vi "NMLWSD_Stability_Data_Collection RevA.vi"(0 "Instrumentation References":T3, 1 "Data Processing":T6, 2 "Tpass Shtr Open":bool, 3 "Log File":path=path "C:/Test/WSNM Stability/Log.txt", 5 "Serial Numbers & COM Ports":T4={"Serial Number"=["1"], "Active UUT COMs"=[]}, 7 "References":T5, 9 "UUT Input Parameters":T2 {"WL: NML Only" items=["Red Only", "IR"]; "FW inTest" items=["WSD Board", "NML Board"]}, 11 "Error In":errorcluster, 12 "Data Results In":T7 {"All Results In" format="%8_4g"}, 13 "Shtr Ctrl Close (s)":dbl=6.0 max=60.0 format="%.3f") -> (4 "Data Results Out":T8 {"All Results Out" format="%8_4g"}, 8 "Data Time":timestamp, 10 "Shtr Ref Time":timestamp, 15 "Error Out":errorcluster)   [LabVIEW 2017]
uses:
  C:/Program Files (x86)/Newport/Newport USB Driver/Bin/UsbDllWrap.dll
  Program Files (x86)/Newport/Newport USB Driver/Bin/UsbDllWrap.dll
  <vilib>/Analysis/baseanly.llb/Mean (DBL).vi
  <vilib>/Utility/file.llb/Write Delimited Spreadsheet (string).vi
  <vilib>/Analysis/NI_AALBase.lvlib
panel:
  in  "Tab Control":T1(tab)
  out "Error Log Msg":string
  out "Timeout":bool
  out "Data Errors":bool
  out "Module Errors":bool[](array[boolean])
  out "Msg":string="\n\r" caption="Status"
  out "Shtr Open":bool
  out "Shtr Close":bool
  out "read buffer":string
  out "MCU Data":dbl[](array[numeric]) format="%#_5p"
  out "System Data":dbl[](array[numeric]) format="%#_5p"
  out "UUT Download Buffer":string
  out "UUT Count":i32=1
  out "Bytes Rcvd":u32
  out "DateS":string caption="Date"
  out "TimeS":string caption="Time"
  out "MCUTrue":bool[][](array[boolean])
  out "SysTrue":bool[][](array[boolean])
  out "MCUCheck":string[][](array[string])
  out "SysCheck":string[][](array[string])
  out "Points":i32[](array[numeric])
  out "All Results Out":dbl[][][](array[numeric]) format="%8_4g"
  out "MCU Data Array":dbl[][](array[numeric])
  out "System Data Array":dbl[][](array[numeric])
  out "Module Error":refnum<vi>
  out "Read Buffer":refnum<vi>
  out "Error Log":refnum<vi>
  out "Data Error":refnum<vi>
  out "TimeOut Error":refnum<vi>
  out "Status Msg":refnum<vi>
  out "Shutter Closed":refnum<vi>
  out "Shutter Opened":refnum<vi>
  # "Indicators Passed To Calling VI via Control RefNum"
  # "Indicators With Data to be Passed to Calling VI Directly But Grouped Into Single Cluster"
  # "Indicators Passed to Calling VI Directly"
  # "Indicators Used To Store & Process Temporary Data for Each UUT"
  # "Indicators That Provide Information Not Necessary for Calling VI"
  # "Indicators Replicated in \"Data Results Out\" Output Cluster To Be Passed to Calling VI Via RefNum"
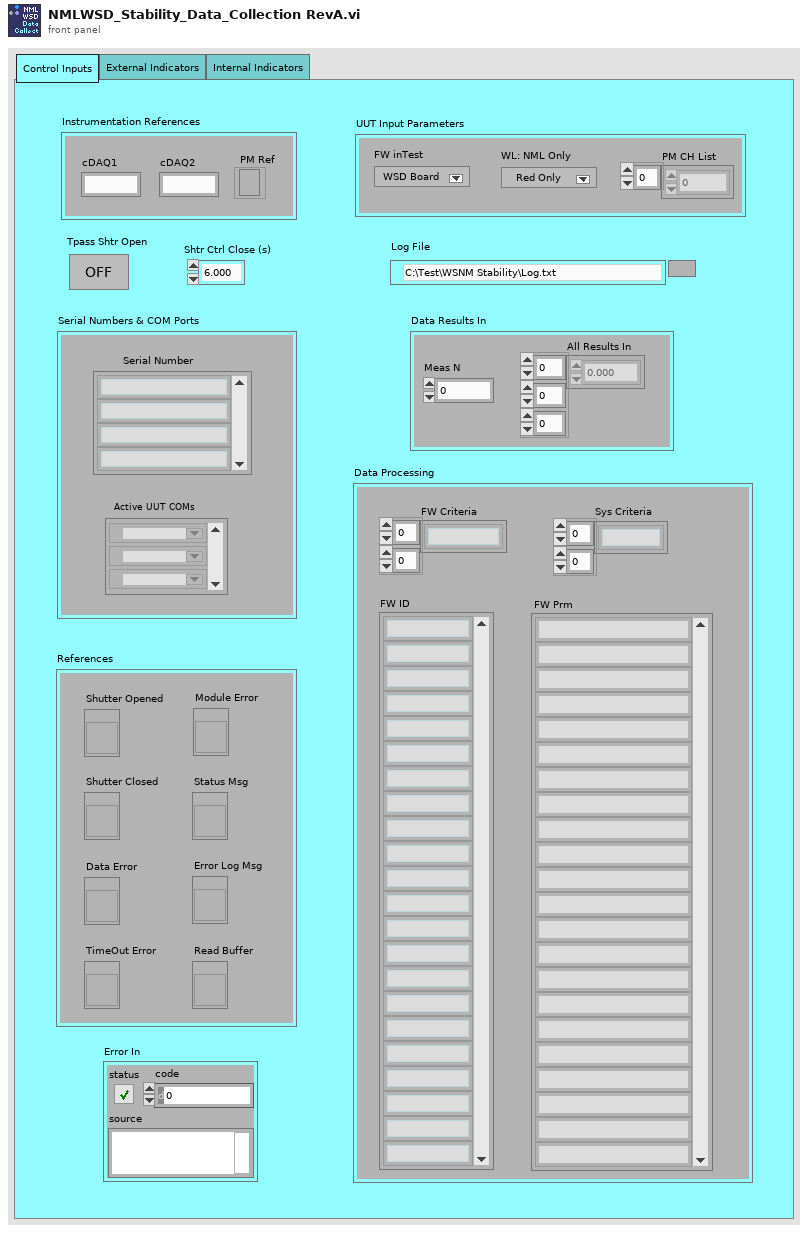
[diagram p1: front panel]
types:
  T1 = enum32{"Control Inputs", "External Indicators", "Internal Indicators"}
  T2 = cluster{"FW inTest":u16, "WL: NML Only":i32, "PM CH List":i32[]}
  T3 = cluster{"cDAQ1":string, "cDAQ2":string, "PM Ref":refnum<k24>}
  T4 = cluster{"Serial Number":string[], "Active UUT COMs":refnum<visa-resource-name>[]}
  T5 = cluster{"Shutter Opened":refnum<vi>, "Shutter Closed":refnum<vi>, "Status Msg":refnum<vi>, "TimeOut Error":refnum<vi>, "Data Error":refnum<vi>, "Error Log Msg":refnum<vi>, "Read Buffer":refnum<vi>, "Module Error":refnum<vi>}
  T6 = cluster{"FW Prm":string[], "FW ID":string[], "FW Criteria":string[][], "Sys Criteria":string[][]}
  T7 = cluster{"Meas N":i32, "All Results In":dbl[][][]}
  T8 = cluster{"MCUTrue":bool[][], "SysTrue":bool[][], "MCUCheck":string[][], "SysCheck":string[][], "Points":i32[], "All Results Out ":dbl[][][], "MCU Data Array":dbl[][], "System Data Array":dbl[][]}
  T9 = cluster{"MCUTrue":bool[][], "SysTrue":bool[][], "MCUCheck":string[][], "SysCheck":string[][], "Points":i32[], "All Results ":dbl[][][], "MCU Data Array":dbl[][], "System Data Array":dbl[][]}
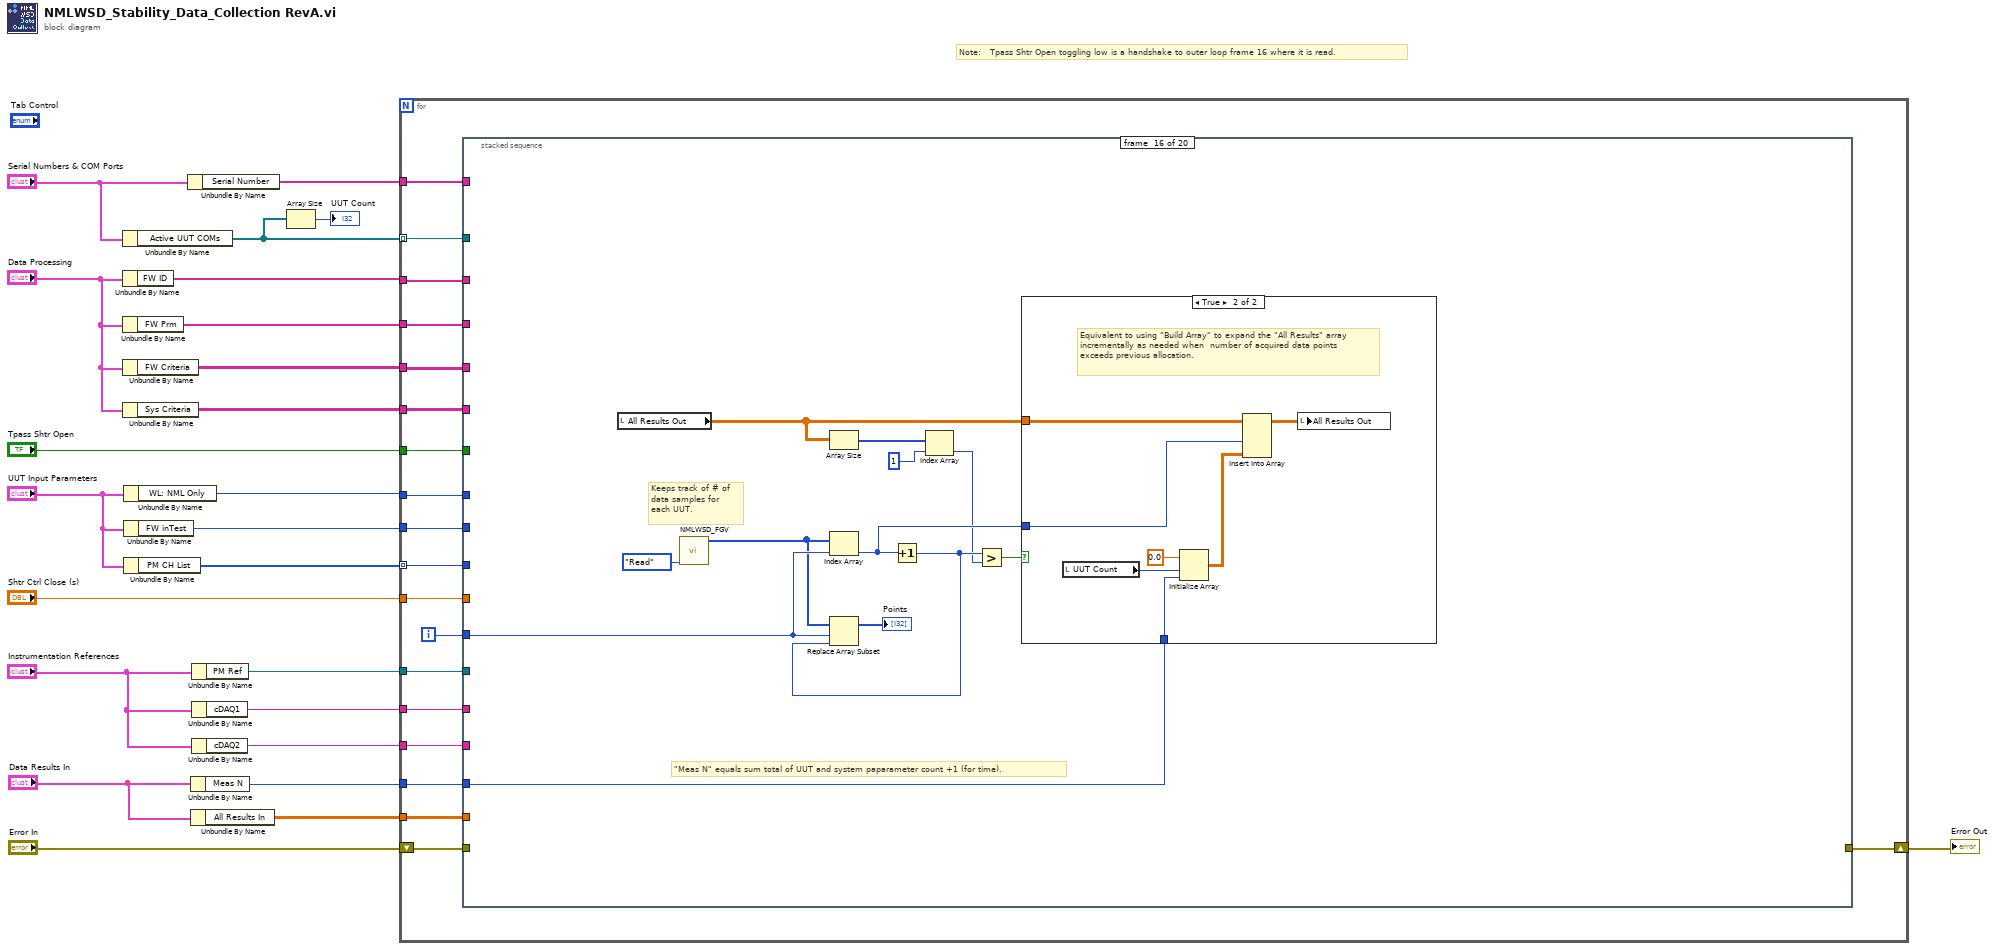
[diagram p0: block diagram]
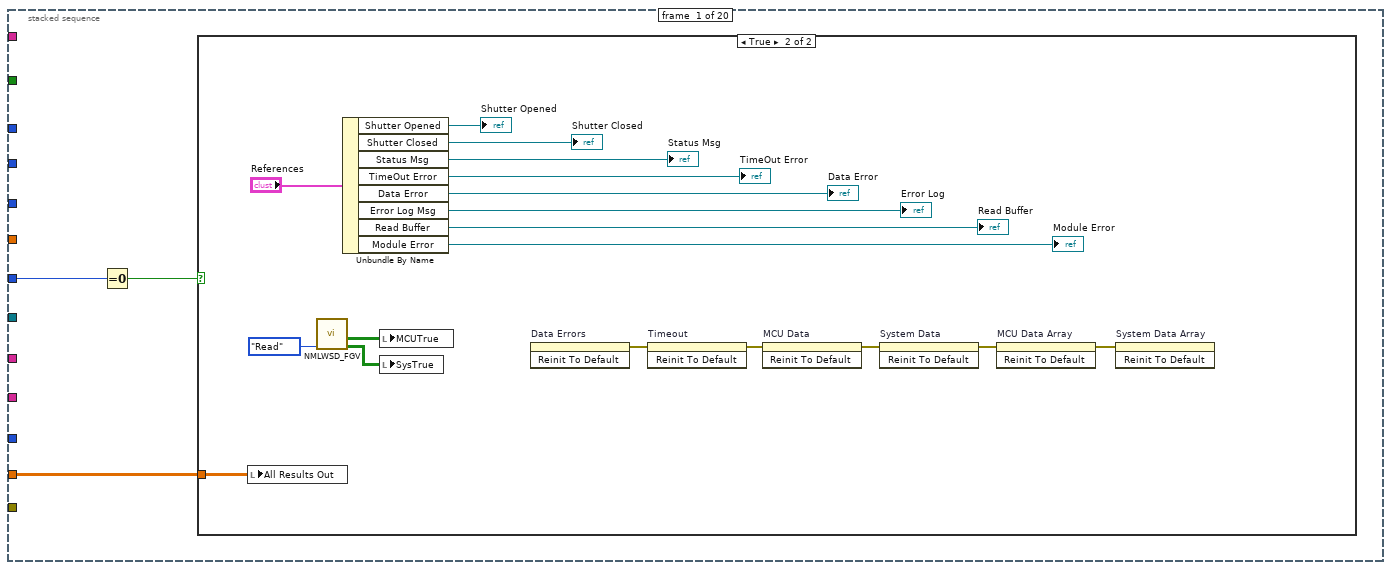
[diagram p2: hidden frame]
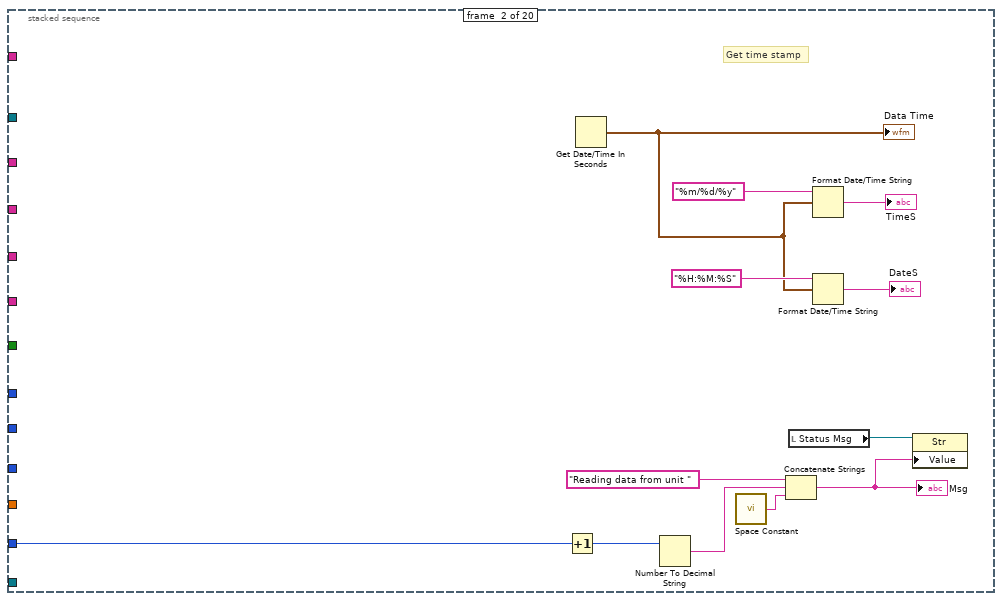
[diagram p4: hidden frame]
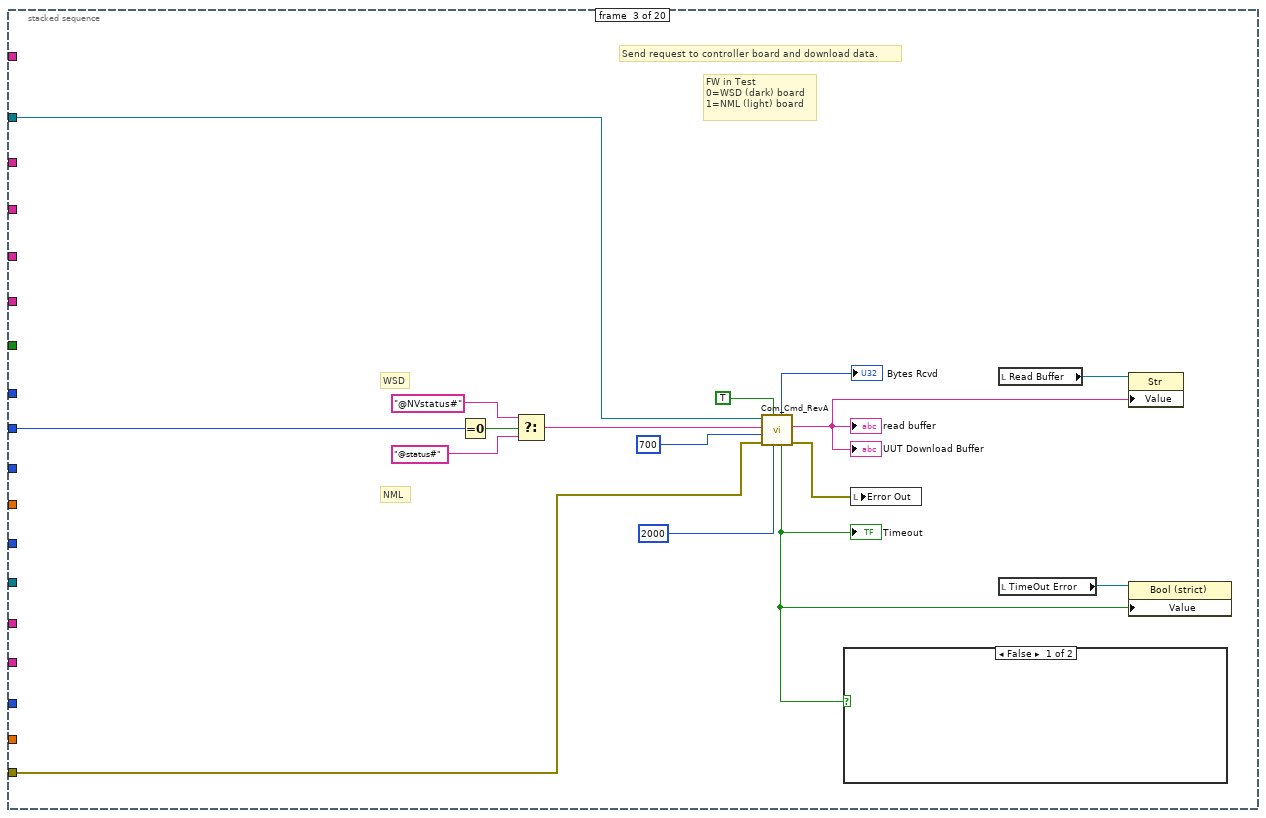
[diagram p5: hidden frame]
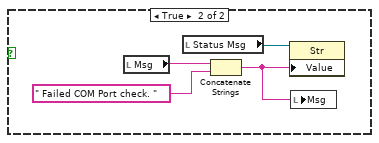
[diagram p6: hidden frame]
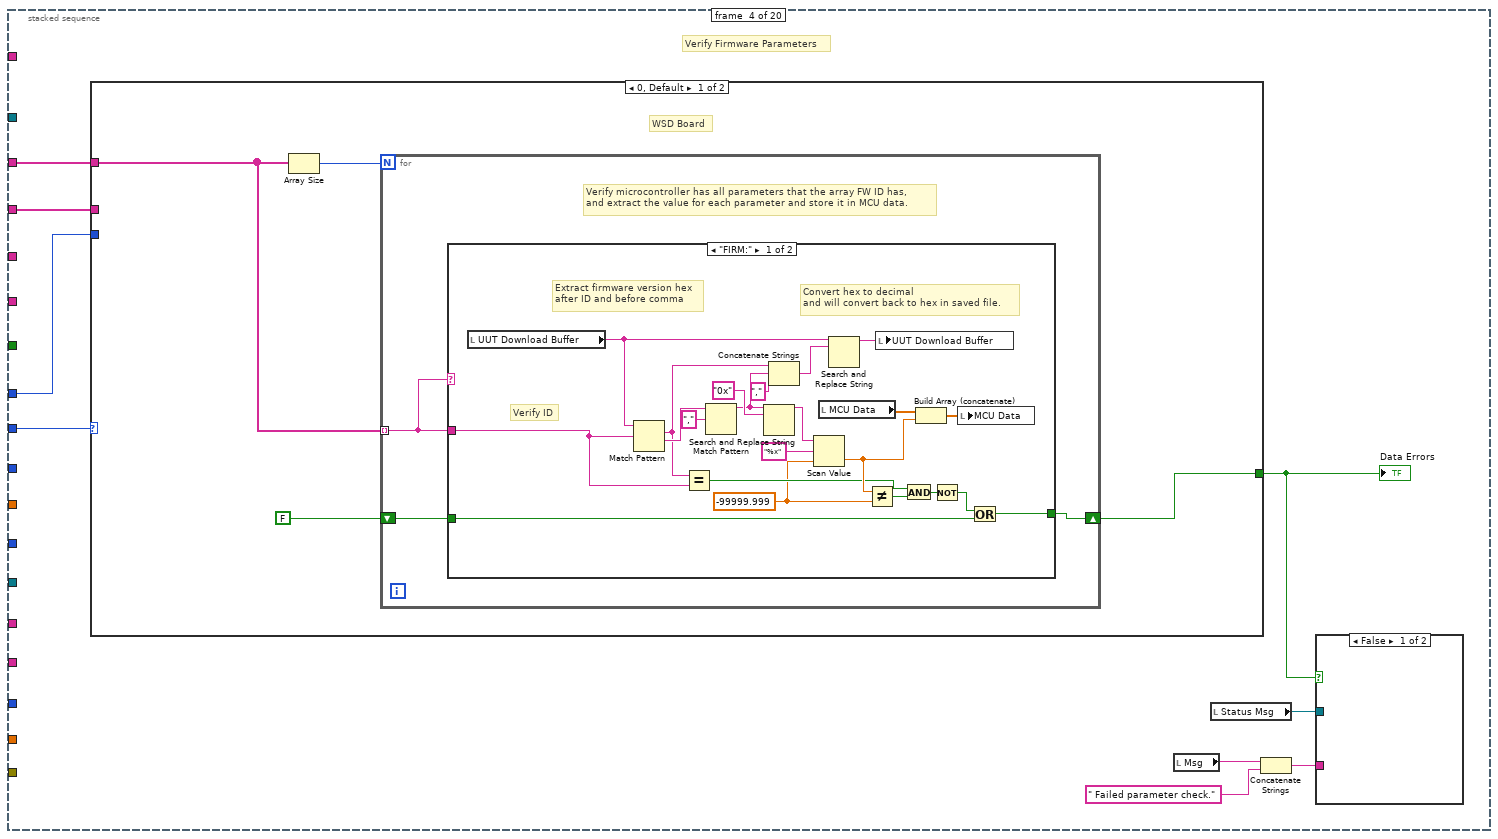
[diagram p7: hidden frame]
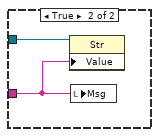
[diagram p8: hidden frame]
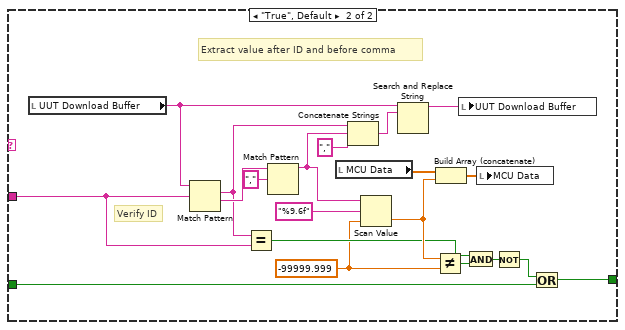
[diagram p9: hidden frame]
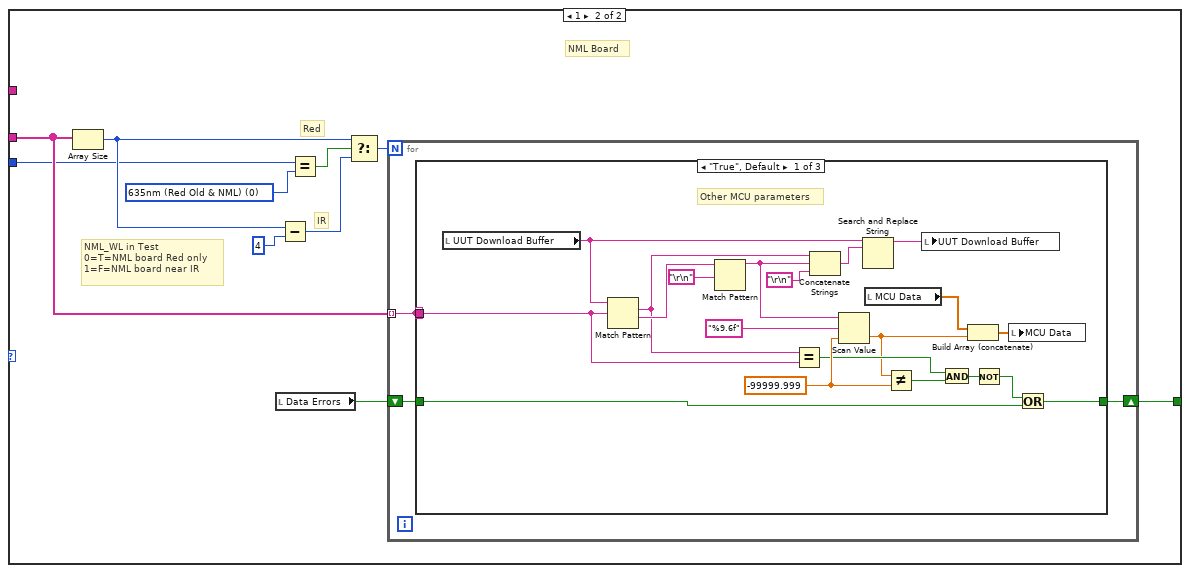
[diagram p10: hidden frame]
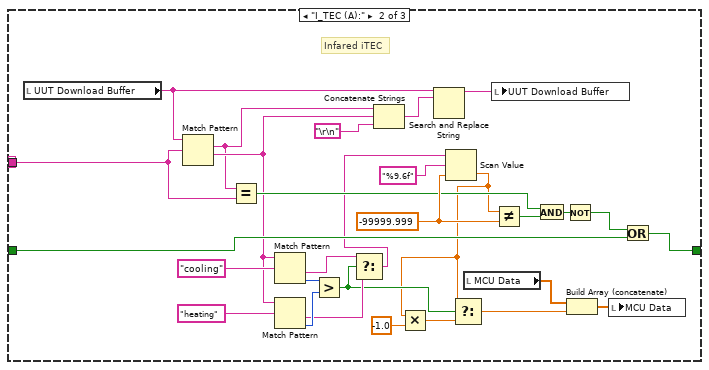
[diagram p11: hidden frame]
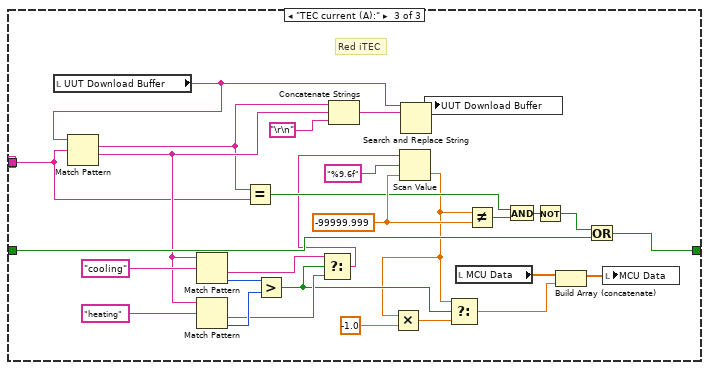
[diagram p12: hidden frame]
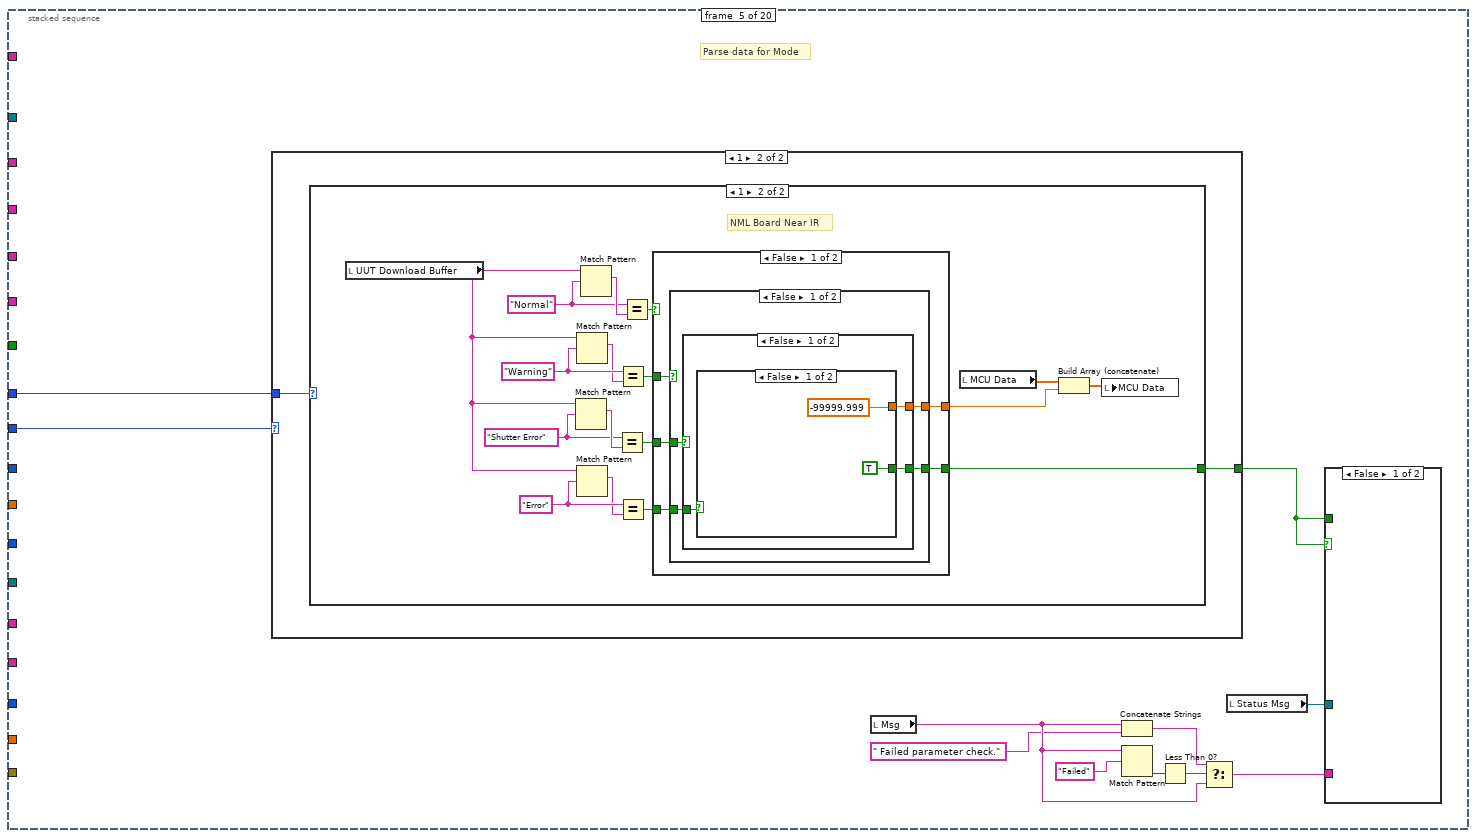
[diagram p13: hidden frame]
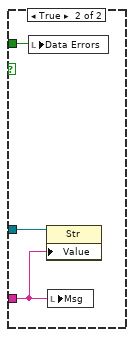
[diagram p14: hidden frame]
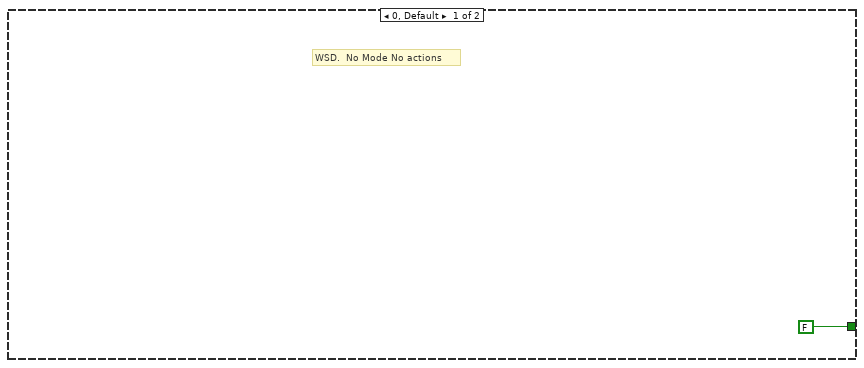
[diagram p15: hidden frame]
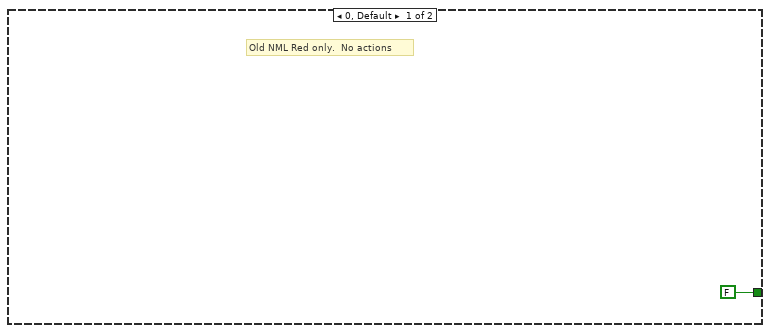
[diagram p16: hidden frame]
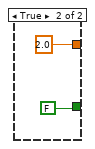
[diagram p17: hidden frame]
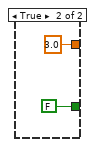
[diagram p18: hidden frame]
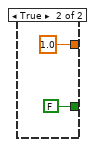
[diagram p19: hidden frame]
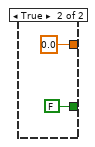
[diagram p20: hidden frame]
diagram:
  # "Note:   Tpass Shtr Open toggling low is a handshake to outer loop frame 16 where it is read."
  n1 = Unbundle By Name("Serial Numbers & COM Ports") -> ("Active UUT COMs"=w13:refnum<visa-resource-name>[])
  n2 = Unbundle By Name("Data Processing") -> ("FW ID"=w12:string[])
  n3 = Unbundle By Name("Data Processing") -> ("FW Prm"=w11:string[])
  n4 = Unbundle By Name("Data Processing") -> ("FW Criteria"=w10:string[][])
  n5 = Unbundle By Name("Data Processing") -> ("Sys Criteria"=w8:string[][])
  n6 = Unbundle By Name("UUT Input Parameters") -> ("WL: NML Only"=w21:i32)
  n7 = Unbundle By Name("UUT Input Parameters") -> ("FW inTest"=w20:u16)
  n8 = Unbundle By Name("UUT Input Parameters") -> ("PM CH List"=w1:i32[])
  n9 = Unbundle By Name("Serial Numbers & COM Ports") -> ("Serial Number"=w14:string[])
  n10 = Unbundle By Name("Data Results In") -> ("Meas N"=w7:i32)
  n11 = Unbundle By Name("Data Results In") -> ("All Results In"=w5:dbl[][][])
  n12 = Unbundle By Name("Instrumentation References") -> ("PM Ref"=w19:refnum<k24>)
  n13 = Unbundle By Name("Instrumentation References") -> ("cDAQ1"=w17:string)
  n14 = Unbundle By Name("Instrumentation References") -> ("cDAQ2"=w16:string)
  n15 = Array Size(array=w13) -> (size(s)=→"UUT Count":i32)
  n16 = for {
    tunnel: w13 -> [w42] mode=indexing
    tunnel: w19 -> [w41]
    tunnel: "Tpass Shtr Open" -> [w40]
    tunnel: w20 -> [w39]
    tunnel: w21 -> [w38]
    tunnel: "Shtr Ctrl Close (s)" -> [w37]
    tunnel: w17 -> [w36]
    tunnel: w16 -> [w35]
    tunnel: w12 -> [w34]
    tunnel: w7 -> [w33]
    tunnel: w14 -> [w32]
    tunnel: w8 -> [w31]
    tunnel: w10 -> [w30]
    tunnel: w11 -> [w29]
    tunnel: w5 -> [w28]
    shift-right: [w26] -> w3
    shift-left: "Error In" -> [w27]
    tunnel: w1 -> [w25] mode=indexing
    i -> [w43]
    n17 = stacked-sequence {
      tunnel: w43 -> [w45 w65 _ _ _ _ _ w412 _ _ _ _ _ w517 w587 w698 w720 w730 w771 w795]
      tunnel: w42 -> [_ _ w85 _ _ _ _ _ _ _ _ _ _ _ _ _ _ _ _ _]
      tunnel: w41 -> [_ _ _ _ _ _ _ _ _ w461 _ _ _ _ w593 _ _ _ _ _]
      tunnel: w40 -> [_ _ _ _ _ _ _ _ _ _ _ _ _ _ w592 _ _ _ _ _]
      tunnel: w39 -> [_ _ w81 w105 w258 w315 w372 _ _ _ _ _ _ _ _ _ _ _ _ _]
      tunnel: w38 -> [_ _ _ w98 w257 w314 w371 _ _ _ _ _ _ _ _ _ _ _ _ _]
      tunnel: w37 -> [_ _ _ _ _ _ _ _ _ _ _ _ _ _ w591 _ _ _ _ _]
      tunnel: w36 -> [_ _ _ _ _ _ _ _ _ _ _ w489 _ w516 w590 _ _ _ _ _]
      tunnel: w35 -> [_ _ _ _ _ _ _ _ _ _ _ _ _ w515 w589 _ _ _ _ _]
      tunnel: w34 -> [_ _ _ w104 _ _ _ _ _ _ _ _ _ _ _ _ _ _ _ _]
      tunnel: w33 -> [_ _ _ _ _ _ _ _ _ _ _ _ _ _ _ w697 _ _ _ _]
      tunnel: w32 -> [_ _ _ _ _ _ _ w410 _ _ _ _ _ _ _ _ _ _ _ _]
      tunnel: w31 -> [_ _ _ _ _ _ _ _ _ _ _ _ _ _ _ _ _ w729 _ _]
      tunnel: w30 -> [_ _ _ _ _ _ _ _ _ _ _ _ _ _ _ _ _ w728 _ _]
      tunnel: w29 -> [_ _ _ w99 _ _ _ _ _ _ _ _ _ _ _ _ _ _ _ _]
      tunnel: w28 -> [w44 _ _ _ _ _ _ _ _ _ _ _ _ _ _ _ _ _ _ _]
      tunnel: w27 -> [_ _ w78 _ _ _ _ _ _ _ _ _ _ _ _ _ _ _ _ _]
      tunnel: [_ _ _ _ _ _ _ _ _ w460 _ _ _ _ _ _ _ _ _ _] -> w26
      tunnel: w25 -> [_ _ _ _ _ _ _ _ _ w459 _ _ _ _ w588 _ _ _ _ _]
      frame #0 {
        n18 = Equal To 0?(x=w45) -> (x = 0?=w46:bool)
        n19 = case shown="True" w46 {
          tunnel: w44 -> [_ w52]
          frame False {
          }
          frame True {
            n20 = local write "All Results Out"(w52) -> ()
            n21 = call "NMLWSD_FGV.vi"("Action"=enum16{"Initialize", "Read", "Write"}."Read") -> ("SysTrue"=w51:bool[][], "MCUTrue"=w50:bool[][])  [unwired: 8 in, 1 out]
            n22 = Unbundle By Name("References") -> ("Shutter Opened"=→"Shutter Opened":refnum<vi>, "Shutter Closed"=→"Shutter Closed":refnum<vi>, "Status Msg"=→"Status Msg":refnum<vi>, "TimeOut Error"=→"TimeOut Error":refnum<vi>, "Data Error"=→"Data Error":refnum<vi>, "Error Log Msg"=→"Error Log":refnum<vi>, "Read Buffer"=→"Read Buffer":refnum<vi>, "Module Error"=→"Module Error":refnum<vi>)
            n23 = local write "MCUTrue"(w50) -> ()
            n24 = local write "SysTrue"(w51) -> ()
            n25 = invoke on="Data Errors" class="Bool (strict)" method="Reinit To Default"() -> (error out=w63:errorcluster)  [unwired: 3 in, 2 out]
            n26 = invoke on="Timeout" class="Bool (strict)" method="Reinit To Default"(error in=w63) -> (error out=w62:errorcluster)  [unwired: 2 in, 2 out]
            n27 = invoke on="MCU Data" class="Arr (strict)" method="Reinit To Default"(error in=w62) -> (error out=w64:errorcluster)  [unwired: 2 in, 2 out]
            n28 = invoke on="System Data" class="Arr (strict)" method="Reinit To Default"(error in=w64) -> (error out=w48:errorcluster)  [unwired: 2 in, 2 out]
            n29 = invoke on="MCU Data Array" class="Arr (strict)" method="Reinit To Default"(error in=w48) -> (error out=w47:errorcluster)  [unwired: 2 in, 2 out]
            n30 = invoke on="System Data Array" class="Arr (strict)" method="Reinit To Default"(error in=w47) -> ()  [unwired: 2 in, 3 out]
          }
        }
      }
      frame #1 {
        # "Get time stamp"
        n31 = Increment(x=w65) -> (x+1=w71:i32)
        n32 = Get Date/Time In Seconds() -> (seconds since 1Jan1904=w72:timestamp)
        "Data Time" <- w72
        n33 = Number To Decimal String(number=w71) -> (decimal integer string=w70:string)  [unwired: 1 in]
        n34 = call <vilib>:"Space Constant.vi"() -> ("String"=w68:string)
        n35 = Concatenate Strings("Reading data from unit " ("Msg"), w70, w68) -> (w69:string)
        "Msg" <- w69
        n36 = local read "Status Msg"() -> (w67:refnum<vi>)
        n37 = Format Date/Time String(time format string (%c)="%m/%d/%y", seconds (now)=w72) -> (date/time string=→"TimeS":string)  [unwired: 1 in]
        n38 = Format Date/Time String(time format string (%c)="%H:%M:%S", seconds (now)=w72) -> (date/time string=→"DateS":string)  [unwired: 1 in]
        n39 = property class="Str"(reference=w67, "Value"=w69) -> ()  [unwired: 1 in, 2 out]
      }
      frame #2 {
        # "NML"
        # "WSD"
        # "FW in Test\n0=WSD (dark) board\n1=NML (light) board"
        # "Send request to controller board and download data."
        n40 = Equal To 0?(x=w81) -> (x = 0?=w86:bool)
        n41 = Select(t="@NVstatus#" ("string"), s=w86, f="@status#" ("string")) -> (s? t:f=w89:string)
        n42 = call "Com_Cmd_RevA.vi"("Timeout"=2000, "Query"=TRUE, "error in"=w78, "Delay, ms"=u32 700, "write buffer"=w89, "VISA"=w85) -> ("error out"=w77:errorcluster, "read buffer"=w83:string, "Timeout"=w84:bool, "return count"=→"Bytes Rcvd":u32)  [unwired: 2 out]
        "UUT Download Buffer" <- w83
        "Timeout" <- w84
        "read buffer" <- w83
        n43 = case shown="False" w84 {
          frame False {
          }
          frame True {
            n44 = local read "Msg"() -> (w96:string)
            n45 = local read "Status Msg"() -> (w93:refnum<vi>)
            n46 = Concatenate Strings(w96, " Failed COM Port check. " ("string")) -> (w94:string)
            n47 = property class="Str"(reference=w93, "Value"=w94) -> ()  [unwired: 1 in, 2 out]
            n48 = local write "Msg"(w94) -> ()
          }
        }
        n49 = local write "Error Out"(w77) -> ()
        n50 = local read "Read Buffer"() -> (w79:refnum<vi>)
        n51 = local read "TimeOut Error"() -> (w80:refnum<vi>)
        n52 = property class="Str"(reference=w79, "Value"=w83) -> ()  [unwired: 1 in, 2 out]
        n53 = property class="Bool (strict)"(reference=w80, "Value"=w84) -> ()  [unwired: 1 in, 2 out]
      }
      frame #3 {
        # "Verify Firmware Parameters"
        n54 = case shown="0, Default" w105 {
          tunnel: w104 -> [w109 _]
          tunnel: [w108 w159] -> w103
          tunnel: w99 -> [_ w158]
          tunnel: w98 -> [_ w157]
          frame 0, Default {
            # "WSD Board"
            n55 = Array Size(array=w109) -> (size(s)=w110:i32)
            n56 = for {
              N: w110 -> [_]
              shift-right: [w113] -> w108
              shift-left: FALSE ("Data Err") -> [w114]
              tunnel: w109 -> [w112] mode=indexing
              # "Verify microcontroller has all parameters that the array FW ID has,\nand extract the value for each parameter and store it in MCU data."
              n57 = case shown="\"FIRM:\"" w112 {
                tunnel: w112 -> [w115 w137]
                tunnel: w114 -> [w125 w156]
                tunnel: [w124 w155] -> w113
                frame "FIRM:" {
                  w129 = -99999.999 ("default (0 dbl)")
                  # "Convert hex to decimal\nand will convert back to hex in saved file."
                  # "Extract firmware version hex\nafter ID and before comma"
                  # "Verify ID"
                  n58 = local read "UUT Download Buffer"() -> (w119:string)
                  n59 = Match Pattern(string=w119, regular expression=w115) -> (match substring=w116:string, after substring=w127:string)  [unwired: 1 in, 2 out]
                  n60 = Equal?(x=w116, y=w115) -> (x = y?=w131:bool)
                  n61 = Match Pattern(string=w127, regular expression=",") -> (before substring=w121:string)  [unwired: 1 in, 3 out]
                  n62 = Search and Replace String(input string=w121, search string="0x") -> (result string=w122:string)  [unwired: 6 in, 3 out]
                  n63 = Concatenate Strings(w116, w121, "," ("string")) -> (w118:string)
                  n64 = Scan Value(string=w122, format string="%x", default (0 dbl)=w129) -> (value=w134:dbl)  [unwired: 1 out]
                  n65 = local read "MCU Data"() -> (w132:dbl[])
                  n66 = Search and Replace String(input string=w119, search string=w118) -> (result string=w117:string)  [unwired: 6 in, 3 out]
                  n67 = Not Equal?(x=w134, y=w129) -> (x != y?=w130:bool)
                  n68 = local write "UUT Download Buffer"(w117) -> ()
                  n69 = And(x=w131, y=w130) -> (x .and. y?=w135:bool)
                  n70 = Build Array (concatenate)(w132, w134) -> (w133:dbl[])
                  n71 = Not(x=w135) -> (.not. x?=w136:bool)
                  n72 = local write "MCU Data"(w133) -> ()
                  n73 = Or(x=w136, y=w125) -> (x .or. y?=w124:bool)
                }
                frame "True", Default {
                  w147 = -99999.999 ("default (0 dbl)")
                  # "Extract value after ID and before comma"
                  # "Verify ID"
                  n74 = local read "UUT Download Buffer"() -> (w141:string)
                  n75 = Match Pattern(string=w141, regular expression=w137) -> (match substring=w138:string, after substring=w145:string)  [unwired: 1 in, 2 out]
                  n76 = Equal?(x=w138, y=w137) -> (x = y?=w149:bool)
                  n77 = Match Pattern(string=w145, regular expression=",") -> (before substring=w142:string)  [unwired: 1 in, 3 out]
                  n78 = local read "MCU Data"() -> (w150:dbl[])
                  n79 = Concatenate Strings(w138, w142, "," ("string")) -> (w140:string)
                  n80 = Scan Value(string=w142, format string="%9.6f", default (0 dbl)=w147) -> (value=w152:dbl)  [unwired: 1 out]
                  n81 = Search and Replace String(input string=w141, search string=w140) -> (result string=w139:string)  [unwired: 6 in, 3 out]
                  n82 = Not Equal?(x=w152, y=w147) -> (x != y?=w148:bool)
                  n83 = Build Array (concatenate)(w150, w152) -> (w151:dbl[])
                  n84 = local write "UUT Download Buffer"(w139) -> ()
                  n85 = And(x=w149, y=w148) -> (x .and. y?=w153:bool)
                  n86 = local write "MCU Data"(w151) -> ()
                  n87 = Not(x=w153) -> (.not. x?=w154:bool)
                  n88 = Or(x=w154, y=w156) -> (x .or. y?=w155:bool)
                }
              }
            }
          }
          frame 1 {
            w161 = 0 items=["635nm (Red Old & NML)", "Red-780-850nm (IR NewNML FW)", "Mix NML FW"] ("Color")
            # "NML Board"
            # "NML_WL in Test\n0=T=NML board Red only\n1=F=NML board near IR"
            # "IR"
            # "Red"
            n89 = Array Size(array=w158) -> (size(s)=w164:i32)
            n90 = local read "Data Errors"() -> (w160:bool)
            n91 = Subtract(x=w164, y=4) -> (x-y=w162:i32)
            n92 = Equal?(x=w157, y=w161) -> (x = y?=w166:bool)
            n93 = Select(t=w164, s=w166, f=w162) -> (s? t:f=w165:i32)
            n94 = for {
              N: w165 -> [_]
              tunnel: w158 -> [w167] mode=indexing
              shift-right: [w168] -> w159
              shift-left: w160 -> [w169]
              n95 = case shown="\"True\", Default" w167 {
                tunnel: w169 -> [w180 w210 w239]
                tunnel: [w179 w209 w238] -> w168
                tunnel: w167 -> [w171 w190 w220]
                frame "True", Default {
                  w188 = -99999.999 ("default (0 dbl)")
                  # "Other MCU parameters"
                  n96 = local read "UUT Download Buffer"() -> (w170:string)
                  n97 = Match Pattern(string=w170, regular expression=w171) -> (match substring=w172:string, after substring=w177:string)  [unwired: 1 in, 2 out]
                  n98 = Match Pattern(string=w177, regular expression="\r\n") -> (before substring=w175:string)  [unwired: 1 in, 3 out]
                  n99 = Equal?(x=w172, y=w171) -> (x = y?=w186:bool)
                  n100 = Concatenate Strings(w172, w175, "\r\n") -> (w174:string)
                  n101 = Scan Value(string=w175, format string="%9.6f", default (0 dbl)=w188) -> (value=w183:dbl)  [unwired: 1 out]
                  n102 = Search and Replace String(input string=w170, search string=w174) -> (result string=w173:string)  [unwired: 6 in, 3 out]
                  n103 = local read "MCU Data"() -> (w185:dbl[])
                  n104 = Not Equal?(x=w183, y=w188) -> (x != y?=w187:bool)
                  n105 = local write "UUT Download Buffer"(w173) -> ()
                  n106 = And(x=w186, y=w187) -> (x .and. y?=w182:bool)
                  n107 = Build Array (concatenate)(w185, w183) -> (w184:dbl[])
                  n108 = Not(x=w182) -> (.not. x?=w181:bool)
                  n109 = local write "MCU Data"(w184) -> ()
                  n110 = Or(x=w181, y=w180) -> (x .or. y?=w179:bool)
                }
                frame "I_TEC (A):" {
                  w217 = -99999.999 ("default (0 dbl)")
                  # "Infared iTEC"
                  n111 = local read "UUT Download Buffer"() -> (w194:string)
                  n112 = Match Pattern(string=w194, regular expression=w190) -> (match substring=w191:string, after substring=w192:string)  [unwired: 1 in, 2 out]
                  n113 = Equal?(x=w191, y=w190) -> (x = y?=w215:bool)
                  n114 = Match Pattern(string=w192, regular expression="cooling") -> (after substring=w204:string, offset past match=w206:i32)  [unwired: 1 in, 2 out]
                  n115 = Match Pattern(string=w192, regular expression="heating") -> (after substring=w203:string, offset past match=w205:i32)  [unwired: 1 in, 2 out]
                  n116 = Greater?(x=w206, y=w205) -> (0:w202:bool)
                  n117 = Select(t=w204, s=w202, f=w203) -> (s? t:f=w193:string)
                  n118 = Concatenate Strings(w191, w192, "\r\n") -> (w197:string)
                  n119 = Search and Replace String(input string=w194, search string=w197) -> (result string=w196:string)  [unwired: 6 in, 3 out]
                  n120 = Scan Value(string=w193, format string="%9.6f", default (0 dbl)=w217) -> (value=w199:dbl)  [unwired: 1 out]
                  n121 = Multiply(x=w199, y=-1.0) -> (x*y=w200:dbl)
                  n122 = Select(t=w199, s=w202, f=w200) -> (s? t:f=w198:dbl)
                  n123 = local read "MCU Data"() -> (w214:dbl[])
                  n124 = local write "UUT Download Buffer"(w196) -> ()
                  n125 = Not Equal?(x=w199, y=w217) -> (x != y?=w216:bool)
                  n126 = And(x=w215, y=w216) -> (x .and. y?=w212:bool)
                  n127 = Not(x=w212) -> (.not. x?=w211:bool)
                  n128 = Build Array (concatenate)(w214, w198) -> (w213:dbl[])
                  n129 = local write "MCU Data"(w213) -> ()
                  n130 = Or(x=w211, y=w210) -> (x .or. y?=w209:bool)
                }
                frame "TEC current (A):" {
                  w246 = -99999.999 ("default (0 dbl)")
                  # "Red iTEC"
                  n131 = local read "UUT Download Buffer"() -> (w222:string)
                  n132 = Match Pattern(string=w222, regular expression=w220) -> (match substring=w219:string, after substring=w221:string)  [unwired: 1 in, 2 out]
                  n133 = Match Pattern(string=w221, regular expression="cooling") -> (after substring=w233:string, offset past match=w235:i32)  [unwired: 1 in, 2 out]
                  n134 = Match Pattern(string=w221, regular expression="heating") -> (after substring=w232:string, offset past match=w234:i32)  [unwired: 1 in, 2 out]
                  n135 = Equal?(x=w219, y=w220) -> (x = y?=w244:bool)
                  n136 = Greater?(x=w235, y=w234) -> (0:w230:bool)
                  n137 = Select(t=w233, s=w230, f=w232) -> (s? t:f=w231:string)
                  n138 = Concatenate Strings(w219, w221, "\r\n") -> (w225:string)
                  n139 = Scan Value(string=w231, format string="%9.6f", default (0 dbl)=w246) -> (value=w227:dbl)  [unwired: 1 out]
                  n140 = Multiply(x=w227, y=-1.0) -> (x*y=w228:dbl)
                  n141 = Search and Replace String(input string=w222, search string=w225) -> (result string=w224:string)  [unwired: 6 in, 3 out]
                  n142 = local write "UUT Download Buffer"(w224) -> ()
                  n143 = Select(t=w227, s=w230, f=w228) -> (s? t:f=w226:dbl)
                  n144 = local read "MCU Data"() -> (w243:dbl[])
                  n145 = Not Equal?(x=w227, y=w246) -> (x != y?=w245:bool)
                  n146 = And(x=w244, y=w245) -> (x .and. y?=w241:bool)
                  n147 = Not(x=w241) -> (.not. x?=w240:bool)
                  n148 = Build Array (concatenate)(w243, w226) -> (w242:dbl[])
                  n149 = Or(x=w240, y=w239) -> (x .or. y?=w238:bool)
                  n150 = local write "MCU Data"(w242) -> ()
                }
              }
            }
          }
        }
        "Data Errors" <- w103
        n151 = local read "Msg"() -> (w102:string)
        n152 = local read "Status Msg"() -> (w97:refnum<vi>)
        n153 = Concatenate Strings(w102, " Failed parameter check." ("string")) -> (w100:string)
        n154 = case shown="False" w103 {
          tunnel: w97 -> [_ w107]
          tunnel: w100 -> [_ w106]
          frame False {
          }
          frame True {
            n155 = property class="Str"(reference=w107, "Value"=w106) -> ()  [unwired: 1 in, 2 out]
            n156 = local write "Msg"(w106) -> ()
          }
        }
      }
      frame #4 {
        # "Parse data for Mode"
        n157 = case shown="1" w258 {
          tunnel: w257 -> [_ w264]
          tunnel: [FALSE w263] -> w250
          frame 0, Default {
            # "WSD.  No Mode No actions"
          }
          frame 1 {
            n158 = case shown="1" w264 {
              tunnel: [FALSE w266] -> w263
              frame 0, Default {
                # "Old NML Red only.  No actions"
              }
              frame 1 {
                w274 = "Error" ("regular expression")
                w275 = "Shutter Error" ("regular expression")
                w278 = "Warning" ("regular expression")
                w279 = "Normal" ("regular expression")
                # "NML Board Near IR"
                n159 = local read "UUT Download Buffer"() -> (w272:string)
                n160 = Match Pattern(string=w272, regular expression=w275) -> (match substring=w276:string)  [unwired: 1 in, 3 out]
                n161 = Match Pattern(string=w272, regular expression=w278) -> (match substring=w277:string)  [unwired: 1 in, 3 out]
                n162 = Match Pattern(string=w272, regular expression=w274) -> (match substring=w273:string)  [unwired: 1 in, 3 out]
                n163 = Match Pattern(string=w272, regular expression=w279) -> (match substring=w282:string)  [unwired: 1 in, 3 out]
                n164 = Equal?(x=w275, y=w276) -> (x = y?=w268:bool)
                n165 = Equal?(x=w278, y=w277) -> (x = y?=w269:bool)
                n166 = Equal?(x=w274, y=w273) -> (x = y?=w267:bool)
                n167 = Equal?(x=w279, y=w282) -> (x = y?=w271:bool)
                n168 = case shown="False" w271 {
                  tunnel: [w286 0.0] -> w270
                  tunnel: w269 -> [w287 _]
                  tunnel: w268 -> [w285 _]
                  tunnel: w267 -> [w284 _]
                  tunnel: [w283 FALSE] -> w266
                  frame False {
                    n169 = case shown="False" w287 {
                      tunnel: [w290 1.0] -> w286
                      tunnel: w285 -> [w291 _]
                      tunnel: w284 -> [w289 _]
                      tunnel: [w288 FALSE] -> w283
                      frame False {
                        n170 = case shown="False" w291 {
                          tunnel: [w293 3.0] -> w290
                          tunnel: w289 -> [w294 _]
                          tunnel: [w292 FALSE] -> w288
                          frame False {
                            n171 = case shown="False" w294 {
                              tunnel: [-99999.999 ("default (0 dbl)") 2.0] -> w293
                              tunnel: [TRUE ("Data Err") FALSE] -> w292
                              frame False {
                              }
                              frame True {
                              }
                            }
                          }
                          frame True {
                          }
                        }
                      }
                      frame True {
                      }
                    }
                  }
                  frame True {
                  }
                }
                n172 = local read "MCU Data"() -> (w281:dbl[])
                n173 = Build Array (concatenate)(w281, w270) -> (w280:dbl[])
                n174 = local write "MCU Data"(w280) -> ()
              }
            }
          }
        }
        n175 = local read "Msg"() -> (w255:string)
        n176 = Concatenate Strings(w255, " Failed parameter check." ("string")) -> (w254:string)
        n177 = Match Pattern(string=w255, regular expression="Failed") -> (offset past match=w252:i32)  [unwired: 1 in, 3 out]
        n178 = Less Than 0?(x=w252) -> (x < 0?=w253:bool)
        n179 = Select(t=w254, s=w253, f=w255) -> (s? t:f=w256:string)
        n180 = local read "Status Msg"() -> (w248:refnum<vi>)
        n181 = case shown="False" w250 {
          tunnel: w248 -> [_ w261]
          tunnel: w256 -> [_ w260]
          tunnel: w250 -> [_ w259]
          frame False {
          }
          frame True {
            n182 = local write "Data Errors"(w259) -> ()
            n183 = property class="Str"(reference=w261, "Value"=w260) -> ()  [unwired: 1 in, 2 out]
            n184 = local write "Msg"(w260) -> ()
          }
        }
      }
      frame #5 {
        # "Parse data for wavelength."
        n185 = case shown="1" w315 {
          tunnel: w314 -> [_ w321]
          tunnel: [FALSE w320] -> w307
          frame 0, Default {
            # "WSD.  No Mode No actions"
          }
          frame 1 {
            # "NML_WL in Test\n0=T=NML board Red only\n1=F=NML board near IR"
            # "NML"
            n186 = case shown="1" w321 {
              tunnel: [FALSE w323] -> w320
              frame 0, Default {
                # "Old NML Red only.  No actions"
              }
              frame 1 {
                w331 = "850" ("regular expression")
                w332 = "780" ("regular expression")
                w335 = "Red" ("regular expression")
                w336 = "None" ("regular expression")
                # "NML IR"
                n187 = local read "UUT Download Buffer"() -> (w329:string)
                n188 = Match Pattern(string=w329, regular expression=w332) -> (match substring=w333:string)  [unwired: 1 in, 3 out]
                n189 = Match Pattern(string=w329, regular expression=w335) -> (match substring=w334:string)  [unwired: 1 in, 3 out]
                n190 = Match Pattern(string=w329, regular expression=w331) -> (match substring=w330:string)  [unwired: 1 in, 3 out]
                n191 = Match Pattern(string=w329, regular expression=w336) -> (match substring=w339:string)  [unwired: 1 in, 3 out]
                n192 = Equal?(x=w332, y=w333) -> (x = y?=w325:bool)
                n193 = Equal?(x=w335, y=w334) -> (x = y?=w326:bool)
                n194 = Equal?(x=w331, y=w330) -> (x = y?=w324:bool)
                n195 = Equal?(x=w336, y=w339) -> (x = y?=w328:bool)
                n196 = case shown="False" w328 {
                  tunnel: [w343 0.0] -> w327
                  tunnel: w326 -> [w344 _]
                  tunnel: w325 -> [w342 _]
                  tunnel: w324 -> [w341 _]
                  tunnel: [w340 FALSE] -> w323
                  frame False {
                    n197 = case shown="False" w344 {
                      tunnel: [w347 1.0] -> w343
                      tunnel: w342 -> [w348 _]
                      tunnel: w341 -> [w346 _]
                      tunnel: [w345 FALSE] -> w340
                      frame False {
                        n198 = case shown="False" w348 {
                          tunnel: [w350 2.0] -> w347
                          tunnel: w346 -> [w351 _]
                          tunnel: [w349 FALSE] -> w345
                          frame False {
                            n199 = case shown="False" w351 {
                              tunnel: [-99999.999 ("default (0 dbl)") 3.0] -> w350
                              tunnel: [TRUE ("Data Err") FALSE] -> w349
                              frame False {
                              }
                              frame True {
                              }
                            }
                          }
                          frame True {
                          }
                        }
                      }
                      frame True {
                      }
                    }
                  }
                  frame True {
                  }
                }
                n200 = local read "MCU Data"() -> (w338:dbl[])
                n201 = Build Array (concatenate)(w338, w327) -> (w337:dbl[])
                n202 = local write "MCU Data"(w337) -> ()
              }
            }
          }
        }
        n203 = local read "Msg"() -> (w309:string)
        n204 = Concatenate Strings(w309, " Failed parameter check." ("string")) -> (w310:string)
        n205 = Match Pattern(string=w309, regular expression="Failed") -> (offset past match=w313:i32)  [unwired: 1 in, 3 out]
        n206 = Less Than 0?(x=w313) -> (x < 0?=w311:bool)
        n207 = Select(t=w310, s=w311, f=w309) -> (s? t:f=w308:string)
        n208 = local read "Status Msg"() -> (w305:refnum<vi>)
        n209 = case shown="False" w307 {
          tunnel: w305 -> [_ w318]
          tunnel: w308 -> [_ w317]
          tunnel: w307 -> [_ w316]
          frame False {
          }
          frame True {
            n210 = local write "Data Errors"(w316) -> ()
            n211 = property class="Str"(reference=w318, "Value"=w317) -> ()  [unwired: 1 in, 2 out]
            n212 = local write "Msg"(w317) -> ()
          }
        }
      }
      frame #6 {
        # "Parse Data for LHM Calibration Gain and Offset"
        n213 = case shown="1" w372 {
          tunnel: w371 -> [_ w378]
          tunnel: [FALSE w377] -> w364
          frame 0, Default {
            # "WSD.  No Mode No actions"
          }
          frame 1 {
            # "NML"
            n214 = case shown="1" w378 {
              tunnel: [FALSE w381] -> w377
              frame 0, Default {
                # "Old NML Red only.  No actions"
              }
              frame 1 {
                w382 = "LHM Calibration:" ("regular expression")
                w389 = -99999.999 ("default (0 dbl)")
                # "NML IR"
                n215 = local read "UUT Download Buffer"() -> (w396:string)
                n216 = Match Pattern(string=w396, regular expression=w382) -> (match substring=w383:string, after substring=w397:string)  [unwired: 1 in, 2 out]
                n217 = Equal?(x=w383, y=w382) -> (x = y?=w401:bool)
                n218 = Match Pattern(string=w397, regular expression="Gain=") -> (after substring=w392:string)  [unwired: 1 in, 3 out]
                n219 = Match Pattern(string=w397, regular expression="Offset=") -> (after substring=w393:string)  [unwired: 1 in, 3 out]
                n220 = Match Pattern(string=w392, regular expression=",") -> (before substring=w391:string)  [unwired: 1 in, 3 out]
                n221 = Concatenate Strings(w383, w397, "\r\n") -> (w399:string)
                n222 = Search and Replace String(input string=w396, search string=w399) -> (result string=w398:string)  [unwired: 6 in, 3 out]
                n223 = Scan Value(string=w391, format string="%9.6f", default (0 dbl)=w389) -> (value=w403:dbl)  [unwired: 1 out]
                n224 = Scan Value(string=w393, format string="%9.6f", default (0 dbl)=w389) -> (value=w404:dbl)  [unwired: 1 out]
                n225 = Not Equal?(x=w403, y=w389) -> (x != y?=w402:bool)
                n226 = local write "UUT Download Buffer"(w398) -> ()
                n227 = Not Equal?(x=w404, y=w389) -> (x != y?=w395:bool)
                n228 = Compound Arithmetic op=AND(w401, w402, w395) -> (w394:bool)
                n229 = Not(x=w394) -> (.not. x?=w381:bool)
                n230 = local read "MCU Data"() -> (w400:dbl[])
                n231 = Build Array (concatenate)(w400, w403, w404) -> (→"MCU Data":dbl[])
              }
            }
          }
        }
        n232 = local read "Msg"() -> (w367:string)
        n233 = Concatenate Strings(w367, " Failed parameter check." ("string")) -> (w368:string)
        n234 = Match Pattern(string=w367, regular expression="Failed") -> (offset past match=w370:i32)  [unwired: 1 in, 3 out]
        n235 = Less Than 0?(x=w370) -> (x < 0?=w369:bool)
        n236 = local read "Status Msg"() -> (w362:refnum<vi>)
        n237 = Select(t=w368, s=w369, f=w367) -> (s? t:f=w366:string)
        n238 = case shown="False" w364 {
          tunnel: w362 -> [_ w375]
          tunnel: w366 -> [_ w374]
          tunnel: w364 -> [_ w373]
          frame False {
          }
          frame True {
            n239 = local write "Data Errors"(w373) -> ()
            n240 = property class="Str"(reference=w375, "Value"=w374) -> ()  [unwired: 1 in, 2 out]
            n241 = local write "Msg"(w374) -> ()
          }
        }
      }
      frame #7 {
        # "Log error if COM port timeout or data error occurs."
        n242 = local read "Timeout"() -> (w411:bool)
        n243 = local read "Data Errors"() -> (w408:bool)
        n244 = Index Array(array=w410, index=w412) -> (element=w420:string)
        n245 = local read "Data Error"() -> (w406:refnum<vi>)
        n246 = Select(t=" Data Corrupted" ("Msg"), s=w408, f=" Data Received" ("Msg")) -> (s? t:f=w422:string)
        n247 = Select(t=" No Response at COM port" ("Msg"), s=w411, f=w422) -> (s? t:f=w418:string)
        n248 = Concatenate Strings("Unit " ("Msg"), w420) -> (w419:string)
        n249 = property class="Bool (strict)"(reference=w406, "Value"=w408) -> ()  [unwired: 1 in, 2 out]
        n250 = Concatenate Strings(w419, w418) -> (w409:string)
        n251 = Concatenate Strings(w409, "\r\n") -> (w414:string)
        n252 = Or(x=w411, y=w408) -> (x .or. y?=w413:bool)
        n253 = case shown="True" w413 {
          tunnel: w414 -> [_ w433]
          tunnel: w412 -> [w425 w432]
          tunnel: [w424 w429] -> w407
          frame False {
            n254 = local read "Module Errors"() -> (w427:bool[])
            n255 = Replace Array Subset(array=w427, new element=FALSE ("new element/subarray"), index=w425) -> (w424:bool[])
          }
          frame True {
            w434 = "\t"
            w439 = "" ("replace string (\"\")")
            w440 = "\r\n"
            n256 = Get Date/Time In Seconds() -> (seconds since 1Jan1904=w448:timestamp)
            n257 = Format Date/Time String(time format string (%c)="%m/%d/%y", seconds (now)=w448) -> (date/time string=w442:string)  [unwired: 1 in]
            n258 = Format Date/Time String(time format string (%c)="%H:%M:%S", seconds (now)=w448) -> (date/time string=w441:string)  [unwired: 1 in]
            n259 = local read "Module Errors"() -> (w444:bool[])
            n260 = local read "Error Log Msg"() -> (w451:string)
            n261 = Search and Replace String(input string=w442, search string=w440, replace string=w439) -> (result string=w436:string)  [unwired: 5 in, 3 out]
            n262 = Search and Replace String(input string=w441, search string=w440, replace string=w439) -> (result string=w435:string)  [unwired: 5 in, 3 out]
            n263 = Build Array(w436, w434, w435, w434, w433) -> (w437:string[])
            n264 = Replace Array Subset(array=w444, new element=TRUE ("new element/subarray"), index=w432) -> (w429:bool[])
            n265 = local read "Error Log"() -> (w428:refnum<vi>)
            n266 = Concatenate Strings(w451, w437) -> (w430:string)
            "Error Log Msg" <- w430
            n267 = Wait Until Next ms Multiple(millisecond multiple=u32 300) -> ()  [unwired: 1 out]
            n268 = property class="Str"(reference=w428, "Value"=w430) -> ()  [unwired: 1 in, 2 out]
            n269 = call-poly <vilib>:"Write Delimited Spreadsheet.vi"("file path (dialog if empty)"="Log File", "1D data"=w437, "append to file? (new file:F)"=TRUE ("transpose? (no:F)"), "transpose? (no:F)"=TRUE ("append to file? (new file:F)"), "delimiter (\\t)"="," ("delimiter (\\t)")) -> ()  [unwired: 9 in, 2 out]
          }
        }
        "Module Errors" <- w407
        n270 = local read "Module Error"() -> (w405:refnum<vi>)
        n271 = property class="Arr (strict)"(reference=w405, "Value"=w407) -> ()  [unwired: 1 in, 2 out]
      }
      frame #8 {
        n272 = local read "Msg"() -> (w456:string)
        n273 = Match Pattern(string=w456, regular expression="Failed") -> (offset past match=w455:i32)  [unwired: 1 in, 3 out]
        n274 = Greater Than 0?(x=w455) -> (x > 0?=w454:bool)
        n275 = Select(t=w456, s=w454, f="Reading Power Meter" ("Msg")) -> (s? t:f=w458:string)
        n276 = local read "Status Msg"() -> (w452:refnum<vi>)
        n277 = property class="Str"(reference=w452, "Value"=w458) -> ()  [unwired: 1 in, 2 out]
        n278 = local write "Msg"(w458) -> ()
      }
      frame #9 {
        # "Channel Select"
        # "Ch2"
        # "Ch1"
        # "Read PM"
        n279 = local read "Error Out"() -> (w480:errorcluster)
        n280 = Quotient & Remainder(x=w459, y=2) -> (x-y*floor(x/y)=w468:i32, floor(x/y)=w462:i32)
        n281 = Increment(x=w462) -> (x+1=w463:i32)
        n282 = call "NewPort_PM_USB_Read-Set.vi"("reference"=w461, "USB Address"=w463, "Read Power(F)\nSet Lambda(T)"=FALSE ("Read Power(T)\nSet Lambda(F)"), "error in"=w480, "Read Power\nSingle CH(F)\nDual CHs(T)"=TRUE ("Set Lambda\nSingle CH(F)\nDual CHs(T)")) -> ("Query-String Format\nfrom Read Buffer"=w477:string, "error out"=w460:errorcluster)  [unwired: 9 in]
        n283 = Number To Boolean Array(number=w468) -> (Boolean array=w467:bool[])
        n284 = Index Array(array=w467, index=0) -> (element=w465:bool)
        n285 = Match Pattern(string=w477, regular expression=",") -> (before substring=w476:string, after substring=w475:string)  [unwired: 1 in, 2 out]
        n286 = Not(x=w465) -> (.not. x?=w464:bool)
        n287 = Fract/Exp String To Number(string=w476) -> (number=w471:dbl)  [unwired: 3 in, 1 out]
        n288 = Fract/Exp String To Number(string=w475) -> (number=w470:dbl)  [unwired: 3 in, 1 out]
        n289 = Select(t=w471, s=w464, f=w470) -> (s? t:f=w472:dbl)
        n290 = local read "System Data"() -> (w481:dbl[])
        n291 = Build Array (concatenate)(w481, w472) -> (w473:dbl[])
        n292 = local write "System Data"(w473) -> ()
      }
      frame #10 {
        n293 = local read "Msg"() -> (w487:string)
        n294 = Match Pattern(string=w487, regular expression="Failed") -> (offset past match=w486:i32)  [unwired: 1 in, 3 out]
        n295 = Greater Than 0?(x=w486) -> (x > 0?=w485:bool)
        n296 = Select(t=w487, s=w485, f="Reading Temperature" ("Msg")) -> (s? t:f=w488:string)
        n297 = local read "Status Msg"() -> (w482:refnum<vi>)
        n298 = property class="Str"(reference=w482, "Value"=w488) -> ()  [unwired: 1 in, 2 out]
        n299 = local write "Msg"(w488) -> ()
      }
      frame #11 {
        # "Get Temp"
        n300 = Concatenate Strings(w489, "Mod4" ("string")) -> (w490:string)
        n301 = call "DAQ Assistant"("device name"=w490) -> ("data"=w492:dynamicdata)  [unwired: 16 in, 2 out]
        n302 = Split Signals(w492) -> (w499:dynamicdata, w497:dynamicdata, w496:dynamicdata, w491:dynamicdata)  [unwired: 4 in]
        n303 = call "Convert from Dynamic Data"("Dynamic Data Type"=w499) -> ("Array"=w498:dbl[])  [unwired: 3 in]
        n304 = call "Convert from Dynamic Data2"("Dynamic Data Type"=w497) -> ("Array"=w495:dbl[])  [unwired: 3 in]
        n305 = call "Convert from Dynamic Data3"("Dynamic Data Type"=w496) -> ("Array"=w494:dbl[])  [unwired: 3 in]
        n306 = call "Convert from Dynamic Data4"("Dynamic Data Type"=w491) -> ("Array"=w493:dbl[])  [unwired: 3 in]
        n307 = call-poly <vilib>:"Mean.vi"("X"=w498) -> ("mean"=w504:dbl)  [unwired: 1 out]
        n308 = call-poly <vilib>:"Mean.vi"("X"=w495) -> ("mean"=w503:dbl)  [unwired: 1 out]
        n309 = call-poly <vilib>:"Mean.vi"("X"=w494) -> ("mean"=w502:dbl)  [unwired: 1 out]
        n310 = call-poly <vilib>:"Mean.vi"("X"=w493) -> ("mean"=w501:dbl)  [unwired: 1 out]
        n311 = local read "System Data"() -> (w506:dbl[])
        n312 = Build Array (concatenate)(w506, w504, w503, w502, w501) -> (w505:dbl[])
        n313 = local write "System Data"(w505) -> ()
      }
      frame #12 {
        n314 = local read "Msg"() -> (w512:string)
        n315 = Match Pattern(string=w512, regular expression="Failed") -> (offset past match=w511:i32)  [unwired: 1 in, 3 out]
        n316 = Greater Than 0?(x=w511) -> (x > 0?=w510:bool)
        n317 = Select(t=w512, s=w510, f="Reading DAQ data" ("Msg")) -> (s? t:f=w513:string)
        n318 = local read "Status Msg"() -> (w507:refnum<vi>)
        n319 = property class="Str"(reference=w507, "Value"=w513) -> ()  [unwired: 1 in, 2 out]
        n320 = local write "Msg"(w513) -> ()
      }
      frame #13 {
        # "Get DAQ data"
        n321 = case shown="0, Default" w517 {
          tunnel: [w558 w562 w564 w568 w574 w578 w580 w584] -> w535
          tunnel: w516 -> [w555 w559 w563 w567 _ _ _ _]
          tunnel: w515 -> [_ _ _ _ w571 w575 w579 w583]
          frame 0, Default {
            n322 = Concatenate Strings(w555, "Mod3" ("string")) -> (w556:string)
            n323 = call "DAQ Assistant2"("device name"=w556) -> ("data"=w558:dynamicdata)  [unwired: 16 in, 2 out]
          }
          frame 1 {
            n324 = Concatenate Strings(w559, "Mod3" ("string")) -> (w560:string)
            n325 = call "DAQ Assistant3"("device name"=w560) -> ("data"=w562:dynamicdata)  [unwired: 16 in, 2 out]
          }
          frame 2 {
            n326 = Concatenate Strings(w563, "Mod2" ("string")) -> (w565:string)
            n327 = call "DAQ Assistant4"("device name"=w565) -> ("data"=w564:dynamicdata)  [unwired: 16 in, 2 out]
          }
          frame 3 {
            n328 = Concatenate Strings(w567, "Mod2" ("string")) -> (w569:string)
            n329 = call "DAQ Assistant5"("device name"=w569) -> ("data"=w568:dynamicdata)  [unwired: 16 in, 2 out]
          }
          frame 4 {
            n330 = Concatenate Strings(w571, "Mod3" ("string")) -> (w572:string)
            n331 = call "DAQ Assistant6"("device name"=w572) -> ("data"=w574:dynamicdata)  [unwired: 16 in, 2 out]
          }
          frame 5 {
            n332 = Concatenate Strings(w575, "Mod3" ("string")) -> (w576:string)
            n333 = call "DAQ Assistant7"("device name"=w576) -> ("data"=w578:dynamicdata)  [unwired: 16 in, 2 out]
          }
          frame 6 {
            n334 = Concatenate Strings(w579, "Mod2" ("string")) -> (w581:string)
            n335 = call "DAQ Assistant8"("device name"=w581) -> ("data"=w580:dynamicdata)  [unwired: 16 in, 2 out]
          }
          frame 7 {
            n336 = Concatenate Strings(w583, "Mod2" ("string")) -> (w585:string)
            n337 = call "DAQ Assistant9"("device name"=w585) -> ("data"=w584:dynamicdata)  [unwired: 16 in, 2 out]
          }
        }
        n338 = Split Signals(w535) -> (w537:dynamicdata, w539:dynamicdata, w540:dynamicdata, w541:dynamicdata, w530:dynamicdata, w527:dynamicdata, w528:dynamicdata, w529:dynamicdata)  [unwired: 8 in]
        n339 = call "Convert from Dynamic Data5"("Dynamic Data Type"=w537) -> ("Array"=w538:dbl[])  [unwired: 3 in]
        n340 = call "Convert from Dynamic Data6"("Dynamic Data Type"=w539) -> ("Array"=w542:dbl[])  [unwired: 3 in]
        n341 = call "Convert from Dynamic Data7"("Dynamic Data Type"=w540) -> ("Array"=w543:dbl[])  [unwired: 3 in]
        n342 = call "Convert from Dynamic Data8"("Dynamic Data Type"=w541) -> ("Array"=w544:dbl[])  [unwired: 3 in]
        n343 = call "Convert from Dynamic Data9"("Dynamic Data Type"=w530) -> ("Array"=w534:dbl[])  [unwired: 3 in]
        n344 = call "Convert from Dynamic Data10"("Dynamic Data Type"=w527) -> ("Array"=w533:dbl[])  [unwired: 3 in]
        n345 = call "Convert from Dynamic Data11"("Dynamic Data Type"=w528) -> ("Array"=w532:dbl[])  [unwired: 3 in]
        n346 = call "Convert from Dynamic Data12"("Dynamic Data Type"=w529) -> ("Array"=w531:dbl[])  [unwired: 3 in]
        n347 = call-poly <vilib>:"Mean.vi"("X"=w538) -> ("mean"=w553:dbl)  [unwired: 1 out]
        n348 = call-poly <vilib>:"Mean.vi"("X"=w542) -> ("mean"=w518:dbl)  [unwired: 1 out]
        n349 = call-poly <vilib>:"Mean.vi"("X"=w543) -> ("mean"=w551:dbl)  [unwired: 1 out]
        n350 = call-poly <vilib>:"Mean.vi"("X"=w544) -> ("mean"=w519:dbl)  [unwired: 1 out]
        n351 = call-poly <vilib>:"Mean.vi"("X"=w534) -> ("mean"=w549:dbl)  [unwired: 1 out]
        n352 = call-poly <vilib>:"Mean.vi"("X"=w533) -> ("mean"=w520:dbl)  [unwired: 1 out]
        n353 = call-poly <vilib>:"Mean.vi"("X"=w532) -> ("mean"=w521:dbl)  [unwired: 1 out]
        n354 = call-poly <vilib>:"Mean.vi"("X"=w531) -> ("mean"=w522:dbl)  [unwired: 1 out]
        n355 = Multiply(x=w518, y=0.25 ("mean")) -> (x*y=w552:dbl)
        n356 = Multiply(x=w519, y=0.25 ("mean")) -> (x*y=w550:dbl)
        n357 = Multiply(x=w520, y=0.25 ("mean")) -> (x*y=w548:dbl)
        n358 = Multiply(x=w521, y=5.814 ("mean")) -> (x*y=w547:dbl)
        n359 = Multiply(x=w522, y=0.25 ("mean")) -> (x*y=w546:dbl)
        n360 = Build Array(w553, w552, w551, w550, w549, w548, w547, w546) -> (w545:dbl[])
        n361 = local read "System Data"() -> (w554:dbl[])
        n362 = Build Array (concatenate)(w554, w545) -> (→"System Data":dbl[])
      }
      frame #14 {
        # "Take optical power readings if shutter open time met minimum duration requirement."
        n363 = case shown="True" w592 {
          tunnel: w593 -> [_ w602]
          tunnel: w591 -> [_ w601]
          tunnel: w590 -> [_ w600]
          tunnel: w589 -> [_ w599]
          tunnel: w588 -> [_ w598]
          tunnel: w587 -> [_ w597]
          frame False {
            # "If required time duration for open shutter not met, use zero value as place holder for closed shutter power reading."
            n364 = local read "System Data"() -> (w594:dbl[])
            n365 = Build Array (concatenate)(w594, 0.0 ("element")) -> (w596:dbl[])
            n366 = local write "System Data"(w596) -> ()
          }
          frame True {
            n367 = stacked-sequence {
              tunnel: w602 -> [_ _ _ w642 _ _]
              tunnel: w601 -> [_ _ w637 _ _ _]
              tunnel: w600 -> [w606 _ _ _ w666 _]
              tunnel: w599 -> [w605 _ _ _ w665 _]
              tunnel: w598 -> [_ _ _ w641 _ _]
              tunnel: w597 -> [w603 _ _ _ _ w681]
              frame #0 {
                w613 = 4 ("y")
                w616 = FALSE
                # "Close shutter individually with respect to the particular unit under test."
                n368 = Build Array(w616, w616, w616, w616) -> (w615:bool[])
                n369 = local read "Msg"() -> (w611:string)
                n370 = Greater Or Equal?(x=w603, y=w613) -> (x >= y?=w614:bool)
                n371 = case shown="True" w614 {
                  tunnel: w603 -> [w620 w627]
                  tunnel: w615 -> [w622 w629]
                  tunnel: w613 -> [w619 _]
                  tunnel: w606 -> [_ w626]
                  tunnel: w605 -> [w617 _]
                  frame True {
                    n372 = Subtract(x=w620, y=w619) -> (x-y=w618:i32)
                    n373 = Replace Array Subset(array=w622, new element=TRUE, index=w618) -> (w621:bool[])
                    n374 = Concatenate Strings(w617, "Mod1" ("string")) -> (w625:string)
                    n375 = call "DAQ Assistant10"("data"=w621, "device name"=w625) -> ()  [unwired: 16 in, 2 out]
                  }
                  frame False {
                    n376 = Replace Array Subset(array=w629, new element=TRUE, index=w627) -> (w628:bool[])
                    n377 = Concatenate Strings(w626, "Mod1" ("string")) -> (w632:string)
                    n378 = call "DAQ Assistant11"("data"=w628, "device name"=w632) -> ()  [unwired: 16 in, 2 out]
                  }
                }
                n379 = Match Pattern(string=w611, regular expression="Failed") -> (offset past match=w610:i32)  [unwired: 1 in, 3 out]
                n380 = Greater Than 0?(x=w610) -> (x > 0?=w609:bool)
                n381 = Select(t=w611, s=w609, f="Cycle shutter to take PM data." ("Msg")) -> (s? t:f=w612:string)
                n382 = local read "Status Msg"() -> (w604:refnum<vi>)
                n383 = property class="Str"(reference=w604, "Value"=w612) -> ()  [unwired: 1 in, 2 out]
                n384 = local write "Msg"(w612) -> ()
              }
              frame #1 {
                w636 = FALSE ("Sttrs Open")
                w635 = TRUE ("Sttrs Close")
                # "Update calling VI indicators"
                # "No need to pass this indicator value to calling VI."
                # "No need to pass this indicator value to calling VI."
                n385 = local read "Shutter Closed"() -> (w634:refnum<vi>)
                n386 = local read "Shutter Opened"() -> (w633:refnum<vi>)
                n387 = property class="Bool (strict)"(reference=w634, "Value"=w635) -> ()  [unwired: 1 in, 2 out]
                n388 = local write "Shtr Close"(w635) -> ()
                n389 = property class="Bool (strict)"(reference=w633, "Value"=w636) -> ()  [unwired: 1 in, 2 out]
                n390 = local write "Shtr Open"(w636) -> ()
              }
              frame #2 {
                # "Close shutter for specified interval."
                n391 = To Unsigned Long Integer(number=w637) -> (unsigned 32bit integer=w638:u32)
                n392 = Multiply(x=w638, y=u32 1000 ("milliseconds to wait")) -> (x*y=w640:u32)
                n393 = Wait (ms)(milliseconds to wait=w640) -> ()  [unwired: 1 out]
              }
              frame #3 {
                # "Channel Select"
                # "Ch2"
                # "Ch1"
                # "USB-read power meter while shutter closed."
                n394 = local read "Error Out"() -> (w662:errorcluster)
                n395 = Quotient & Remainder(x=w641, y=2) -> (x-y*floor(x/y)=w653:i32, floor(x/y)=w644:i32)
                n396 = Increment(x=w644) -> (x+1=w643:i32)
                n397 = call "NewPort_PM_USB_Read-Set.vi"("reference"=w642, "USB Address"=w643, "Read Power(F)\nSet Lambda(T)"=FALSE ("Read Power(T)\nSet Lambda(F)"), "error in"=w662, "Read Power\nSingle CH(F)\nDual CHs(T)"=TRUE ("Set Lambda\nSingle CH(F)\nDual CHs(T)")) -> ("Query-String Format\nfrom Read Buffer"=w661:string, "error out"=w656:errorcluster)  [unwired: 9 in]
                n398 = local write "Error Out"(w656) -> ()
                n399 = Number To Boolean Array(number=w653) -> (Boolean array=w652:bool[])
                n400 = Index Array(array=w652, index=0) -> (element=w651:bool)
                n401 = Match Pattern(string=w661, regular expression=",") -> (before substring=w660:string, after substring=w659:string)  [unwired: 1 in, 2 out]
                n402 = Not(x=w651) -> (.not. x?=w650:bool)
                n403 = Fract/Exp String To Number(string=w660) -> (number=w655:dbl)  [unwired: 3 in, 1 out]
                n404 = Fract/Exp String To Number(string=w659) -> (number=w654:dbl)  [unwired: 3 in, 1 out]
                n405 = Select(t=w655, s=w650, f=w654) -> (s? t:f=w657:dbl)
                n406 = local read "System Data"() -> (w663:dbl[])
                n407 = Build Array (concatenate)(w663, w657) -> (w658:dbl[])
                n408 = local write "System Data"(w658) -> ()
              }
              frame #4 {
                w672 = FALSE
                # "No need to pass this indicator value to calling VI."
                # "No need to pass this indicator value to calling VI."
                # "F=open, T=closed"
                n409 = Build Array(w672, w672, w672, w672) -> (w671:bool[])
                n410 = local read "UUT Count"() -> (w670:i32)
                n411 = Greater?(x=w670, y=4) -> (0:w668:bool)
                n412 = case shown="False" w668 {
                  tunnel: w671 -> [w674 w678]
                  tunnel: w666 -> [_ w677]
                  tunnel: w665 -> [w673 _]
                  frame True {
                    n413 = Concatenate Strings(w673, "Mod1" ("string")) -> (w676:string)
                    n414 = call "DAQ Assistant12"("data"=w674, "device name"=w676) -> ()  [unwired: 16 in, 2 out]
                  }
                  frame False {
                    n415 = Concatenate Strings(w677, "Mod1" ("string")) -> (w680:string)
                    n416 = call "DAQ Assistant13"("data"=w678, "device name"=w680) -> ()  [unwired: 16 in, 2 out]
                  }
                }
                "Shtr Open" <- TRUE ("Sttrs Open")
                "Shtr Close" <- FALSE ("Sttrs Close")
              }
              frame #5 {
                # "Update the start time of shutter open after data collected for all units in this particular sample."
                n417 = local read "UUT Count"() -> (w691:i32)
                n418 = Increment(x=w681) -> (x+1=w689:i32)
                n419 = local read "Msg"() -> (w687:string)
                n420 = Greater Or Equal?(x=w689, y=w691) -> (x >= y?=w690:bool)
                n421 = case shown="True" w690 {
                  frame False {
                  }
                  frame True {
                    # "Not necessary to toggle this Boolean if\nperformed in calling VI after execution."
                    n422 = local read "Data Time"() -> (→"Shtr Ref Time":timestamp)
                    n423 = local write "Tpass Shtr Open"(FALSE ("Pass 3 Minute")) -> ()
                  }
                }
                n424 = Match Pattern(string=w687, regular expression="Failed") -> (offset past match=w686:i32)  [unwired: 1 in, 3 out]
                n425 = Greater Than 0?(x=w686) -> (x > 0?=w685:bool)
                n426 = Select(t=w687, s=w685, f="Save and process collected data." ("Msg")) -> (s? t:f=w688:string)
                n427 = local read "Status Msg"() -> (w682:refnum<vi>)
                n428 = property class="Str"(reference=w682, "Value"=w688) -> ()  [unwired: 1 in, 2 out]
                n429 = local write "Msg"(w688) -> ()
              }
            }
          }
        }
      }
      frame #15 {
        # "\"Meas N\" equals sum total of UUT and system paparameter count +1 (for time)."
        # "Keeps track of # of\ndata samples for\neach UUT."
        n430 = local read "All Results Out"() -> (w702:dbl[][][])
        n431 = call "NMLWSD_FGV.vi"("Action"=enum16{"Initialize", "Read", "Write"}."Read") -> ("Points Read"=w695:i32[])  [unwired: 8 in, 2 out]
        n432 = Array Size(array=w702) -> (size(s)=w699:i32[])
        n433 = Index Array(array=w695, index=w698) -> (element=w705:i32)
        n434 = Increment(x=w705) -> (x+1=w704:i32)
        n435 = Replace Array Subset(array=w695, new element=w704, index=w698) -> (→"Points":i32[])
        n436 = Index Array(array=w699, index=1) -> (element=w701:i32)
        n437 = Greater?(x=w704, y=w701) -> (0:w703:bool)
        n438 = case shown="True" w703 {
          tunnel: w702 -> [_ w712]
          tunnel: w705 -> [_ w711]
          tunnel: w697 -> [_ w706]
          frame False {
          }
          frame True {
            # "Equivalent to using \"Build Array\" to expand the \"All Results\" array incrementally as needed when  number of acquired data points exceeds previous allocation."
            n439 = local read "UUT Count"() -> (w710:i32)
            n440 = Initialize Array(0.0 ("element"), w710, w706) -> (w708:dbl[][])
            n441 = Insert Into Array(array=w712, index (dim 1)=w711, new element=w708) -> (w707:dbl[][][])  [unwired: 2 in]
            n442 = local write "All Results Out"(w707) -> ()
          }
        }
      }
      frame #16 {
        # "Store newly acquired MCU and System Data to All Results Array."
        # "\"All Results\" Local Variable Indice Definition:\n0 = Unit #\n1 = Sample #\n2 = Parameter Values"
        n443 = local read "All Results Out"() -> (w724:dbl[][][])
        n444 = local read "Points"() -> (w725:i32[])
        n445 = local read "Data Time"() -> (w722:timestamp)
        n446 = local read "MCU Data"() -> (w718:dbl[])
        n447 = local read "System Data"() -> (w714:dbl[])
        n448 = To Double Precision Float(number=w722) -> (double precision float=w721:dbl)
        n449 = Index Array(array=w725, index=w720) -> (element=w726:i32)
        n450 = Build Array (concatenate)(w721, w718, w714) -> (w723:dbl[])
        n451 = Decrement(x=w726) -> (x-1=w727:i32)
        n452 = Replace Array Subset(array=w724, new element=w723, index (dim 0)=w720, index (dim 1)=w727) -> (→"All Results Out":dbl[][][])  [unwired: 1 in]
        n453 = local read "MCU Data Array"() -> (w717:dbl[][])
        n454 = local read "System Data Array"() -> (w715:dbl[][])
        n455 = Build Array (concatenate)(w715, w714) -> (→"System Data Array":dbl[][])
        n456 = Build Array (concatenate)(w717, w718) -> (→"MCU Data Array":dbl[][])
      }
      frame #17 {
        # "max"
        # "min"
        # "max"
        # "min"
        # "Criteria check of test data."
        n457 = Index Array(array=w728, index (col)=1 ("disabled index (col)")) -> (element=w739:string[])  [unwired: 1 in]
        n458 = Index Array(array=w728, index (col)=0 ("disabled index (col)")) -> (element=w740:string[])  [unwired: 1 in]
        n459 = Index Array(array=w729, index (col)=1 ("disabled index (col)")) -> (element=w732:string[])  [unwired: 1 in]
        n460 = Index Array(array=w729, index (col)=0 ("disabled index (col)")) -> (element=w731:string[])  [unwired: 1 in]
        n461 = Array Size(array=w732) -> (size(s)=w733:i32)
        n462 = Array Size(array=w739) -> (size(s)=w738:i32)
        n463 = for {
          N: w738 -> [_]
          tunnel: w739 -> [w767] mode=indexing
          tunnel: w740 -> [w765] mode=indexing
          tunnel: w730 -> [w758]
          i -> [w759]
          n464 = local read "MCU Data"() -> (w770:dbl[])
          n465 = local read "MCUTrue"() -> (w757:bool[][])
          n466 = Scan Value(string=w767, format string="%9.6f") -> (value=w766:dbl)  [unwired: 1 in, 1 out]
          n467 = Index Array(array=w770, index=w759) -> (element=w769:dbl)
          n468 = Scan Value(string=w765, format string="%9.6f") -> (value=w763:dbl)  [unwired: 1 in, 1 out]
          n469 = Index Array(array=w757, index (row)=w759, index (col)=w758) -> (element=w762:bool)
          n470 = In Range and Coerce(upper limit=w766, x=w769, lower limit=w763) -> (In Range?=w760:bool)  [unwired: 1 out]
          n471 = And(x=w760, y=w762) -> (x .and. y?=w761:bool)
          n472 = Replace Array Subset(array=w757, new element=w761, index (row)=w759, index (col)=w758) -> (→"MCUTrue":bool[][])
        }
        n473 = for {
          N: w733 -> [_]
          tunnel: w732 -> [w753] mode=indexing
          tunnel: w731 -> [w751] mode=indexing
          tunnel: w730 -> [w743]
          i -> [w744]
          n474 = local read "SysTrue"() -> (w742:bool[][])
          n475 = local read "System Data"() -> (w746:dbl[])
          n476 = Scan Value(string=w753, format string="%9.6f") -> (value=w752:dbl)  [unwired: 1 in, 1 out]
          n477 = Index Array(array=w746, index=w744) -> (element=w755:dbl)
          n478 = Scan Value(string=w751, format string="%9.6f") -> (value=w749:dbl)  [unwired: 1 in, 1 out]
          n479 = Index Array(array=w742, index (row)=w744, index (col)=w743) -> (element=w748:bool)
          n480 = In Range and Coerce(upper limit=w752, x=w755, lower limit=w749) -> (In Range?=w745:bool)  [unwired: 1 out]
          n481 = And(x=w745, y=w748) -> (x .and. y?=w747:bool)
          n482 = Replace Array Subset(array=w742, new element=w747, index (row)=w744, index (col)=w743) -> (→"SysTrue":bool[][])
        }
      }
      frame #18 {
        # "Question for Jie:  Why  use either \"R\" or no string characters for results of MCUCheck and SysCheck?  Why are these indicators needed in addition to the Boolean arrays?"
        # "7-7-17 Added, convert parameter review status from boolean to string"
        n483 = local read "SysTrue"() -> (w775:bool[][])
        n484 = local read "MCUTrue"() -> (w772:bool[][])
        n485 = Index Array(array=w775, index (col)=w771) -> (element=w774:bool[])  [unwired: 1 in]
        n486 = Index Array(array=w772, index (col)=w771) -> (element=w773:bool[])  [unwired: 1 in]
        n487 = for {
          tunnel: w774 -> [w783] mode=indexing
          tunnel: w771 -> [w779]
          i -> [w778]
          n488 = local read "SysCheck"() -> (w780:string[][])
          n489 = Select(t="", s=w783, f="R") -> (s? t:f=w777:string)
          n490 = Replace Array Subset(array=w780, new element=w777, index (row)=w778, index (col)=w779) -> (→"SysCheck":string[][])
        }
        n491 = for {
          tunnel: w773 -> [w785] mode=indexing
          tunnel: w771 -> [w788]
          i -> [w787]
          n492 = local read "MCUCheck"() -> (w789:string[][])
          n493 = Select(t="", s=w785, f="R") -> (s? t:f=w786:string)
          n494 = Replace Array Subset(array=w789, new element=w786, index (row)=w787, index (col)=w788) -> (→"MCUCheck":string[][])
        }
      }
      frame #19 {
        n495 = Increment(x=w795) -> (x+1=w794:i32)
        n496 = local read "UUT Count"() -> (w793:i32)
        n497 = Equal?(x=w793, y=w794) -> (x = y?=w792:bool)
        n498 = case shown="True" w792 {
          frame False {
          }
          frame True {
            w805 = T9 {"MCUTrue"=[], "SysTrue"=[], "MCUCheck"=[], "SysCheck"=[], "Points"=[], "All Results "=[], "MCU Data Array"=[], "System Data Array"=[]}  # Data Results
            n499 = local read "MCUTrue"() -> (w804:bool[][])
            n500 = local read "SysTrue"() -> (w803:bool[][])
            n501 = local read "MCUCheck"() -> (w802:string[][])
            n502 = local read "SysCheck"() -> (w801:string[][])
            n503 = local read "Points"() -> (w800:i32[])
            n504 = local read "All Results Out"() -> (w799:dbl[][][])
            n505 = local read "MCU Data Array"() -> (w798:dbl[][])
            n506 = local read "System Data Array"() -> (w797:dbl[][])
            n507 = Bundle By Name(cluster=w805, "MCUTrue"=w804, "SysTrue"=w803, "MCUCheck"=w802, "SysCheck"=w801, "Points"=w800, "All Results"=w799, "MCU Data Array"=w798, "System Data Array"=w797) -> (→"Data Results Out":T9)
          }
        }
        n508 = local write "Msg"("Idle" ("Msg")) -> ()
      }
    }
  }
  "Error Out" <- w3
